vi "AB_Rename_Source_CORE.vi"(8 "error in (no error)":errorcluster, 9 "New name":string, 10 "Source items in":refnum<class "AB_Source.lvclass">[](array[class]), 11 "Source in":refnum<class "AB_Source.lvclass">) -> (0 "error out":errorcluster, 2 "New name":string, 3 "Source out":refnum<class "AB_Source.lvclass">)   [LabVIEW 2020]
uses:
  <vilib>/AppBuilder/AB_Classes/Source/AB_Source.lvclass
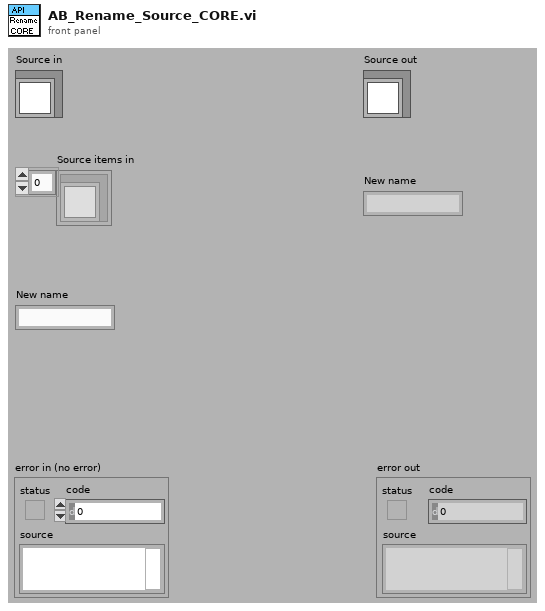
[diagram p1: front panel]
types:
  T1 = typedef "AB_Source.ctl" = cluster{"path":path, "itemID":string, "parentIndex":i32, "sourceInclusion":T2, "destinationIndex":i32, "properties":T3[], "newName":string, "lvfile":bool, "valid":bool, "eng_inBuild":bool, "eng_isNonVILink":bool, "Amalgamation":bool, "Amalgamation Piece":bool, "eng_delimitedName":string, "preventRename":bool}
  T2 = typedef "AB_Source_Inclusion.ctl" = enum16{"IncludeIfReferenced", "Include", "Exclude", "TopLevel"}
  T3 = typedef "AB_Source_Properties.ctl" = cluster{"sourcePropertyType":T4, "value":variant}
  T4 = typedef "AB_Source_Property_Type.ctl" = enum16{"Remove block diagram", "Remove front panel", "Password", "Window has title bar", "Show menu bar", "Show vertical scroll bar", "Show horizontal scroll bar", "Show toolbar", "Show Abort button", "Show fp when called", "Window behavior", "Allow user to close window", "Window run-time position", "Run when opened", "Allow debugging", "Auto error handling", "Generate guard code", "Use stack variables", "Expression folding", "Integer only", "Inline subVI"}
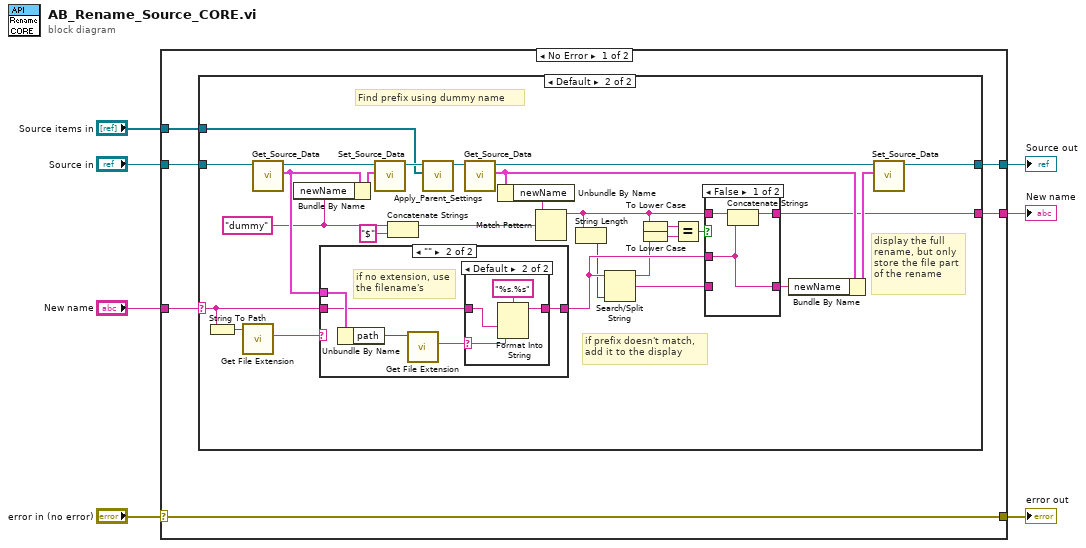
[diagram p0: block diagram]
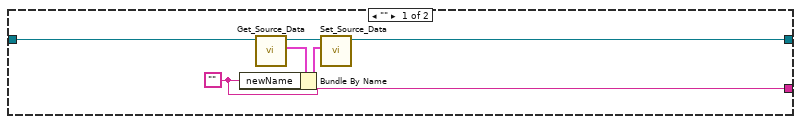
[diagram p2: hidden frame]
diagram:
  n1 = case shown="No Error" "error in (no error)" {
    selector: "error in (no error)" -> [w9 w65]
    tunnel: [w9 w65] -> w6
    tunnel: [w10 _] -> w1
    tunnel: [w13 w64] -> w5
    tunnel: "Source in" -> [w12 w64]
    tunnel: "Source items in" -> [w11 _]
    tunnel: "New name" -> [w8 _]
    frame No Error {
      n2 = case shown="Default" w8 {
        selector: w8 -> [_ w20]
        tunnel: [w15 w24] -> w13
        tunnel: w12 -> [w16 w23]
        tunnel: w11 -> [_ w22]
        tunnel: [w14 w21] -> w10
        frame "" {
          w14 = ""
          n3 = call <vilib>:"Get_Source_Data.vi"("Class in"=w16) -> ("data"=w17:T1, "Class out"=w19:refnum<class "AB_Source.lvclass">)  [unwired: 1 in, 8 out]
          n4 = Bundle By Name(cluster=w17, "newName"=w14) -> (w18:T1)
          n5 = call <vilib>:"Set_Source_Data.vi"("data"=w18, "Class in"=w19) -> ("Class out"=w15:refnum<class "AB_Source.lvclass">)  [unwired: 1 in, 8 out]
        }
        frame Default {
          w34 = "dummy" ("newName")
          # "display the full\nrename, but only\nstore the file part\nof the rename"
          # "if prefix doesn't match,\nadd it to the display"
          # "Find prefix using dummy name"
          n6 = String To Path(string=w20) -> (path=w37:path)
          n7 = call <vilib>:"Get File Extension.vi"("file"=w37) -> ("lowercase file extension"=w36:string)  [unwired: 1 in, 9 out]
          n8 = call <vilib>:"Get_Source_Data.vi"("Class in"=w23) -> ("data"=w35:T1, "Class out"=w32:refnum<class "AB_Source.lvclass">)  [unwired: 1 in, 8 out]
          n9 = Bundle By Name(cluster=w35, "newName"=w34) -> (w31:T1)
          n10 = case shown="\"\"" w36 {
            tunnel: [w48 w50] -> w41
            tunnel: w20 -> [w48 w51]
            tunnel: w35 -> [_ w52]
            frame Default {
            }
            frame "" {
              # "if no extension, use the filename's"
              n11 = Unbundle By Name(w52) -> ("path"=w53:path)
              n12 = call <vilib>:"Get File Extension.vi"("file"=w53) -> ("lowercase file extension"=w49:string)  [unwired: 1 in, 9 out]
              n13 = case shown="Default" w49 {
                selector: w49 -> [_ w55]
                tunnel: w51 -> [w54 w57]
                tunnel: [w54 w56] -> w50
                frame "" {
                  # "unless file had no extension"
                }
                frame Default {
                  n14 = Format Into String(format string="%s.%s", w57, w55) -> (resulting string=w56:string)  [unwired: 2 in, 1 out]
                }
              }
            }
          }
          n15 = call <vilib>:"Set_Source_Data.vi"("data"=w31, "Class in"=w32) -> ("Class out"=w33:refnum<class "AB_Source.lvclass">)  [unwired: 1 in, 8 out]
          n16 = Concatenate Strings(w34, "$" ("string")) -> (w46:string)
          n17 = call-dynamic "Apply_Parent_Settings.vi"("sourceItems in"=w22, "AB_Source in"=w33) -> ("AB_Source out"=w30:refnum<class "AB_Source.lvclass">)  [unwired: 1 in, 8 out]
          n18 = call <vilib>:"Get_Source_Data.vi"("Class in"=w30) -> ("data"=w27:T1, "Class out"=w28:refnum<class "AB_Source.lvclass">)  [unwired: 1 in, 8 out]
          n19 = Unbundle By Name(w27) -> ("newName"=w29:string)
          n20 = Match Pattern(string=w29, regular expression=w46) -> (before substring=w42:string)  [unwired: 4 out]
          n21 = String Length(string=w42) -> (length=w40:i32)
          n22 = Search/Split String(string=w41, offset (0)=w40) -> (substring before match=w39:string, match + rest of string=w38:string)  [unwired: 2 out]
          n23 = To Lower Case(string=w42) -> (all lower case string=w45:string)
          n24 = To Lower Case(string=w39) -> (all lower case string=w44:string)
          n25 = Equal?(x=w45, y=w44) -> (x = y?=w43:bool)
          n26 = case shown="False" w43 {
            tunnel: [w60 w62] -> w21
            tunnel: w42 -> [w61 _]
            tunnel: w41 -> [w59 w62]
            tunnel: [w59 w63] -> w25
            tunnel: w38 -> [_ w63]
            frame False {
              n27 = Concatenate Strings(w61, w59) -> (w60:string)
            }
            frame True {
            }
          }
          n28 = Bundle By Name(cluster=w27, "newName"=w25) -> (w26:T1)
          n29 = call <vilib>:"Set_Source_Data.vi"("data"=w26, "Class in"=w28) -> ("Class out"=w24:refnum<class "AB_Source.lvclass">)  [unwired: 1 in, 8 out]
        }
      }
    }
    frame Error {
    }
  }
  "error out" <- w6
  "Source out" <- w5
  "New name" <- w1
